vi "Queue Command Parse.vi"(11 "command queue datatype":T1) -> (2 "Variant Data":variant, 3 "Command":string)   [LabVIEW 2018]
doc: "Unbundles the Command Q datatype into the Command (String) and the Argument (Variant)\n\n2006 Imaginatics, Mike Ashe\nmichael.ashe@imaginatics.net\nCell: 860-961-0876"
uses:
  Command Queue Cluster.ctl
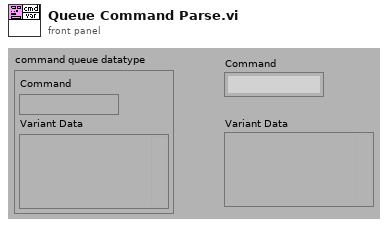
[diagram p1: front panel]
types:
  T1 = typedef "Command Queue Cluster.ctl" = cluster{"Command":string, "Variant Data":variant}
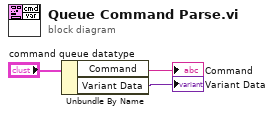
[diagram p0: block diagram]
diagram:
  n1 = Unbundle By Name("command queue datatype") -> ("Command"=→"Command":string, "Variant Data"=→"Variant Data":variant)
